vi "New.vi"(4 "dialog on failure? (T)":bool=TRUE, 5 "minimum log level (Info)":T1=enum."Info", 6 "enabled? (T)":bool=TRUE, 7 "name (\"Default\")":string="Default", 8 "error in (no error)":errorcluster, 9 "log handler (file handler)":refnum<class "Formatting Handler.lvclass">, 10 "log filter (none)":refnum<class "Filter.lvclass">, 11 "logger scope (all)":refnum<class "Scope.lvclass">) -> (0 "error out":errorcluster, 3 "logger":refnum<class "Logger.lvclass">)   [LabVIEW 2018, in "Logging.lvlib" / "Logger.lvclass"]
uses:
  Logger.lvclass
  extension/scope_interface/Scope.lvclass
  extension/formatting_handler_interface/Formatting Handler.lvclass
  extension/filter_interface/Filter.lvclass
  Log Levels.ctl
  Internal Log Levels.ctl
  Logger.lvclass/Logger.ctl
  ae9efc32-4b59-42b1-b54d-2db6c4d58197.vi
  configuration/handlers/file_handler/File Handler.lvclass
  C:/Users/Colin/Documents/software_projects/glog/src/api/extension/formatting_handler_interface/Formatting Handler.lvclass
  <vilib>/Utility/LVClass/Get LV Class Name.vi
  <vilib>/Utility/LVClass/Get LV Class Default Value By Name.vi
  Logging.lvlib
panel:
  # "Connector Pane"
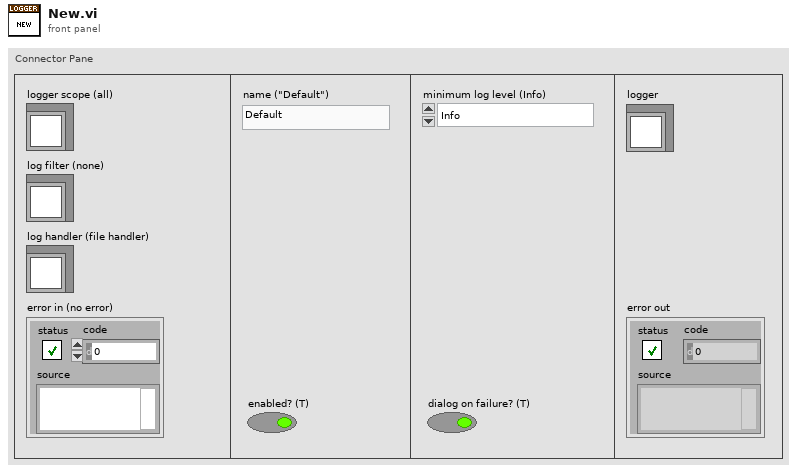
[diagram p1: front panel]
types:
  T1 = typedef "Logging.lvlib/Log Levels.ctl" = enum16{"Trace", "Debug", "Info", "Warning", "Error", "Critical"}
  T2 = typedef "Logging.lvlib/Internal Log Levels.ctl" = enum16{"Trace", "Debug", "Info", "Warning", "Error", "Critical", "Internal"}
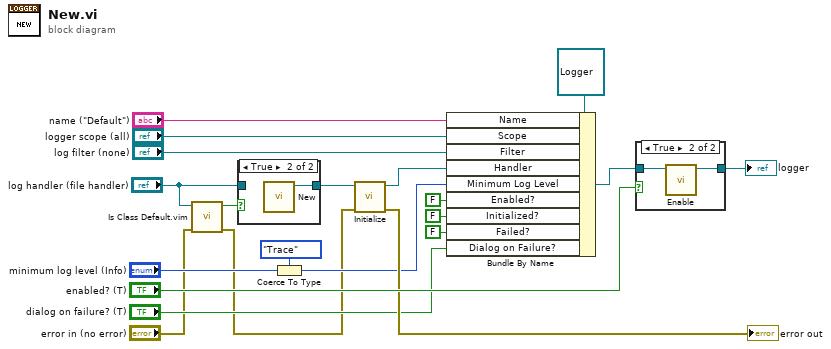
[diagram p0: block diagram]
diagram:
  n1 = call "Is Class Default.vim"("error in (no error)"="error in (no error)", "class"="log handler (file handler)") -> ("error out"=w1:errorcluster, "is default?"=w14:bool)  [unwired: 8 in]
  n2 = case shown="True" w14 {
    tunnel: [w22 w23] -> w17
    tunnel: "log handler (file handler)" -> [w22 _]
    frame False {
    }
    frame True {
      n3 = call "New.vi"() -> ("file handler"=w23:refnum<class "File Handler.lvclass">)  [unwired: 11 in]
    }
  }
  n4 = Coerce To Type(0:"minimum log level (Info)", 1:Internal_Log_Levels."Trace" ("internal log level")) -> (2:w8:T2)
  n5 = call-dynamic "Initialize.vi"("error in (no error)"=w1, "handler in"=w17) -> ("error out"=→"error out":errorcluster, "handler out"=w13:refnum<class "Formatting Handler.lvclass">)  [unwired: 8 in]
  n6 = Bundle By Name(cluster=refnum<class "Logger.lvclass"> refnum ("logger"), "Name"="name (\"Default\")", "Scope"="logger scope (all)", "Filter"="log filter (none)", "Handler"=w13, "Minimum Log Level"=w8, "Enabled?"=FALSE ("Active?"), "Initialized?"=FALSE ("Active?"), "Failed?"=FALSE, "Dialog on Failure?"="dialog on failure? (T)") -> (w6:refnum<class "Logger.lvclass">)
  n7 = case shown="True" "enabled? (T)" {
    tunnel: w6 -> [w24 w26]
    tunnel: [w24 w25] -> w5
    frame False {
    }
    frame True {
      n8 = call "Enable.vi"("logger in"=w26) -> ("logger out"=w25:refnum<class "Logger.lvclass">)  [unwired: 10 in]
    }
  }
  "logger" <- w5
